vi "ThorLab Motor Ctrl.vi"() -> ()   [LabVIEW 2016]
uses:
  <vilib>/platform/TimedLoop/XDataNode/XDataNode.xnode
  <vilib>/Platform/TimedLoop/XDataNode/nitl_modes.ctl
  <vilib>/Platform/TimedLoop/XDataNode/XDNodeRunTimeDep.lvlib
  <vilib>/Platform/TimedLoop/XDataNode/wakeup.ctl
  <vilib>/Platform/TimedLoop/XDataNode/timing_clust.ctl
  <vilib>/rvi/interface/nirviOpenFPGA/nirviOpenFPGA.xnode
  <vilib>/rvi/interface/nirviReadWriteControl/nirviReadWriteControl.xnode
  Library/jmslib.lvlib
  FPGA Bitfiles/IRISSControl_FPGATarget_ThorlabMotorCtrl_umJbgQcQBDg.lvbitx
  Thorlab_MotorCtrl.vi
  <vilib>/FPGAPlugInAG/PXI-7833R/niLvFpga_Open_PXI-7833R.vi
  <vilib>/rvi/interface/common/dynamic/niFpgaDynamicAddResources.vi
  NiFpgaLv.dll
  <vilib>/Utility/error.llb/Error Cluster From Error Code.vi
  <vilib>/rvi/interface/Simulation/niFpgaSimulationCallBeginRW.vi
  <vilib>/rvi/errors/niLvFpgaAdjustHostInterfaceError.vi
panel:
  in  "Motor On":bool=TRUE
  in  "PID Gains":cluster{"Kp":dbl, "Kd":dbl, "Ki":dbl}={"Kp"=0.0001, "Kd"=0.01, "Ki"=0.0}
  in  "Reference Y [mm]":dbl=5.0
  out "Position Y [mm]":dbl
  in  "stop":bool
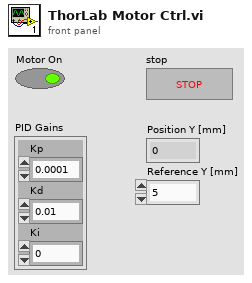
[diagram p1: front panel]
types:
  T1 = typedef "XDNodeRunTimeDep.lvlib/timing_clust.ctl" = cluster{"Expected End [f-1]":u64, "Actual End [f-1]":u64, "Finished Late? [f-1]":bool, "Expected End [i-1]":u64, "Actual End [i-1]":u64, "Finished Late? [i-1]":bool, "Expected Start [i]":u64, "Actual Start [i]":u64, "Expected Start [f]":u64, "Actual Start [f]":u64, "Source Name":string, "Structure Name":string, "Period":i64, "Deadline":i64, "Offset":i64, "Start":i64, "Priority":i32, "Timeout":i32, "Mode":T2, "Wakeup Reason":T3, "Error":errorcluster, "Source Type":string, "Secondary Source Type":string, "Global End Time":u64, "Global Start Time":u64, "Frame Duration":u64, "Iteration Duration":u64, "Assigned CPU":i32, "I/O Scan Engine Mode":u32}
  T2 = typedef "XDNodeRunTimeDep.lvlib/nitl_modes.ctl" = enum32{"No Change", "Process missed periods, maintain original phase", "Discard missed periods, maintain original phase", "Process missed periods, ignore original phase", "Discard missed periods, ignore original phase"}
  T3 = typedef "XDNodeRunTimeDep.lvlib/wakeup.ctl" = enum32{"Normal", "Aborted", "Asynchronous wakeup", "Timing source error", "Timed loop error", "Timeout"}
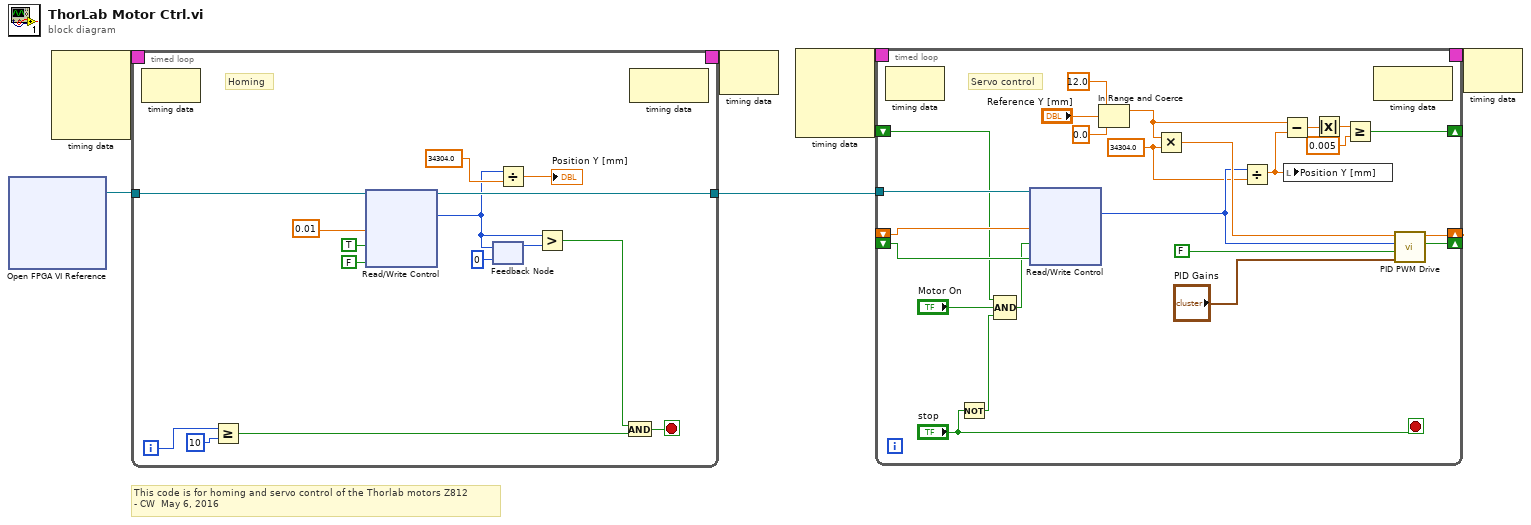
[diagram p0: block diagram]
diagram:
  # "This code is for homing and servo control of the Thorlab motors Z812\n- CW  May 6, 2016"
  n1 = xnode "Open FPGA VI Reference"() -> ("FPGA VI Reference Out"=w2:refnum<k20>)  [unwired: 2 in, 1 out]
  n2 = node-c288() -> (w4:T1)  [unwired: 4 in]
  n3 = timed-loop {
    timing: w4 -> [_]
    timing-out: [_] -> w3
    tunnel: w2 -> [w21]
    tunnel: [w20] -> w1
    i -> [w9]
    stop <- w16 stop-if-true
    # "Homing"
    n4 = node-c288() -> ()  [unwired: 1 in, 1 out]
    n5 = Greater Or Equal?(x=w9, y=10) -> (x >= y?=w7:bool)
    n6 = xnode "Read/Write Control"("FPGA VI Reference In"=w21, "Y DC"=0.01 ("y"), "INHB Y"=TRUE, "DIR Y"=FALSE ("INHB Y")) -> ("FPGA VI Reference Out"=w20:refnum<k20>, "Position Y"=w11:i32)  [unwired: 1 in, 1 out]
    n7 = feedback-in #1(w11) -> ()
    n8 = feedback #1(0 ("Position Y")) -> (w12:i32)
    n9 = Divide(x=w11, y=34304.0) -> (x/y=→"Position Y [mm]":dbl)
    n10 = Greater?(x=w11, y=w12) -> (0:w10:bool)
    n11 = And(x=w10, y=w7) -> (x .and. y?=w16:bool)
    n12 = node-c288() -> ()  [unwired: 1 in, 1 out]
  }
  n13 = node-c288(w3) -> ()  [unwired: 1 out]
  n14 = node-c288() -> (w6:T1)  [unwired: 4 in]
  n15 = timed-loop {
    timing: w6 -> [_]
    timing-out: [_] -> w5
    tunnel: w1 -> [w47]
    shift-right: [w43] -> _
    shift-left: _ -> [w41]
    shift-right: [w42] -> _
    shift-left: _ -> [w40]
    shift-right: [w25] -> _
    shift-left: _ -> [w24]
    stop <- "stop" stop-if-true
    w38 = 34304.0 ("y")
    # "Servo control"
    n16 = node-c288() -> ()  [unwired: 1 in, 1 out]
    n17 = Not(x="stop") -> (.not. x?=w35:bool)
    n18 = Compound Arithmetic op=AND(w24, "Motor On", w35) -> (w34:bool)
    n19 = xnode "Read/Write Control"("FPGA VI Reference In"=w47, "Y DC"=w41, "INHB Y"=w34, "DIR Y"=w40) -> ("Position Y"=w39:i32)  [unwired: 1 in, 2 out]
    n20 = In Range and Coerce(upper limit=12.0, x="Reference Y [mm]", lower limit=0.0) -> (coerced(x)=w30:dbl)  [unwired: 1 out]
    n21 = Multiply(x=w30, y=w38) -> (x*y=w46:dbl)
    n22 = Divide(x=w39, y=w38) -> (x/y=w29:dbl)
    n23 = Subtract(x=w30, y=w29) -> (x-y=w28:dbl)
    n24 = local write "Position Y [mm]"(w29) -> ()
    n25 = Absolute Value(x=w28) -> (abs(x)=w27:dbl)
    n26 = Greater Or Equal?(x=w27, y=0.005) -> (x >= y?=w25:bool)
    n27 = node-c288() -> ()  [unwired: 1 in, 1 out]
    n28 = call "PID PWM Drive.vi"("PID Gains"="PID Gains", "Reverse Motor?"=FALSE, "Encoder Position"=w39, "Reference"=w46) -> ("Direction"=w42:bool, "Duty Cycle"=w43:dbl)  [unwired: 5 in, 1 out]
  }
  n29 = node-c288(w5) -> ()  [unwired: 1 out]
